vi "Import - Rx Packet.vi"(7 "Rx Packet":T1 {"Endianness" items=["big-endian"=0, "little-endian"=2]}, 8 "error in (no error)":errorcluster, 11 "Device Item Ref in":T6 format="%.0x") -> (0 "error out":errorcluster)   [LabVIEW 2016, in "UDP-Custom-Device System Explorer.lvlib"]
uses:
  UDP-Custom-Device System Explorer.lvlib
  <vilib>/NI Veristand/Custom Device API/Custom Device Item Ref.ctl
  Types/XML - New/ImpExp - Rx Packet Data.ctl
  <vilib>/NI Veristand/Custom Device API/Custom Device Item Info.ctl
  Shared/Types/Shared - Channel Data Type.ctl
  Shared/Types/Shared - Buffered.PacketInfo.ctl
  Shared/Types/Shared - Pointer Encoding.ctl
  <vilib>/NI Veristand/Custom Device API/Custom Device Channel.ctl
  <vilib>/NI Veristand/Custom Device API/Custom Device Channel Type.ctl
  Shared/Constants.vi
  Property Accessors/Shared Packet Accessors.lvlib
  Property Accessors/Rx Packet Accessors.lvlib
  <vilib>/NI VeriStand/Custom Device API/Custom Device API.lvlib
  Shared/UDP-Custom-Device Shared.lvlib
  Property Accessors/Rx Channel Accessors.lvlib
  Property Accessors/Rx Channel Section Accessors.lvlib
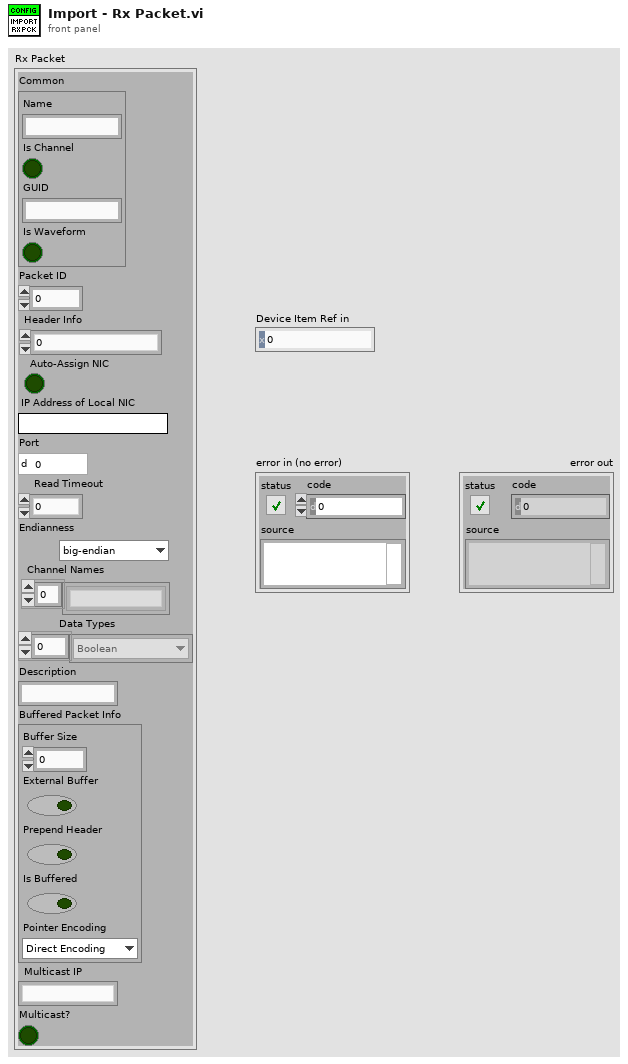
[diagram p1: front panel]
types:
  T1 = typedef "UDP-Custom-Device System Explorer.lvlib/ImpExp - Rx Packet Data.ctl" = cluster{"Common":T2, "Packet ID":i32, "Header Info":u32, "Auto-Assign NIC":bool, "IP Address of Local NIC":string, "Port":u16, "Read Timeout":i32, "Endianness":u16, "Channel Names":string[], "Data Types":T3[], "Description":string, "Buffered Packet Info":T4, "Multicast IP":string, "Multicast?":bool}
  T2 = typedef "Custom Device API.lvlib/Custom Device Item Info.ctl" = cluster{"Name":string, "Is Channel":bool, "GUID":string, "Is Waveform":bool}
  T3 = typedef "UDP-Custom-Device Shared.lvlib/Shared - Channel Data Type.ctl" = enum16{"Boolean", "Single", "Double", "I8", "I16", "I32", "I64", "U8", "U16", "U32", "U64"}
  T4 = typedef "UDP-Custom-Device Shared.lvlib/Shared - Buffered.PacketInfo.ctl" = cluster{"Buffer Size":i32, "External Buffer":bool, "Prepend Header":bool, "Is Buffered":bool, "Pointer Encoding":T5}
  T5 = typedef "UDP-Custom-Device Shared.lvlib/Shared - Pointer Encoding.ctl" = enum16{"Direct Encoding", "Conversion Encoding"}
  T6 = typedef "Custom Device API.lvlib/Custom Device Item Ref.ctl" = u64
  T7 = typedef "Custom Device API.lvlib/Custom Device Channel.ctl" = cluster{"Type":T8, "Units":string, "Default Value":dbl, "Faultable":bool, "Scalable":bool}
  T8 = typedef "Custom Device API.lvlib/Custom Device Channel Type.ctl" = enum16{"Input", "Output"}
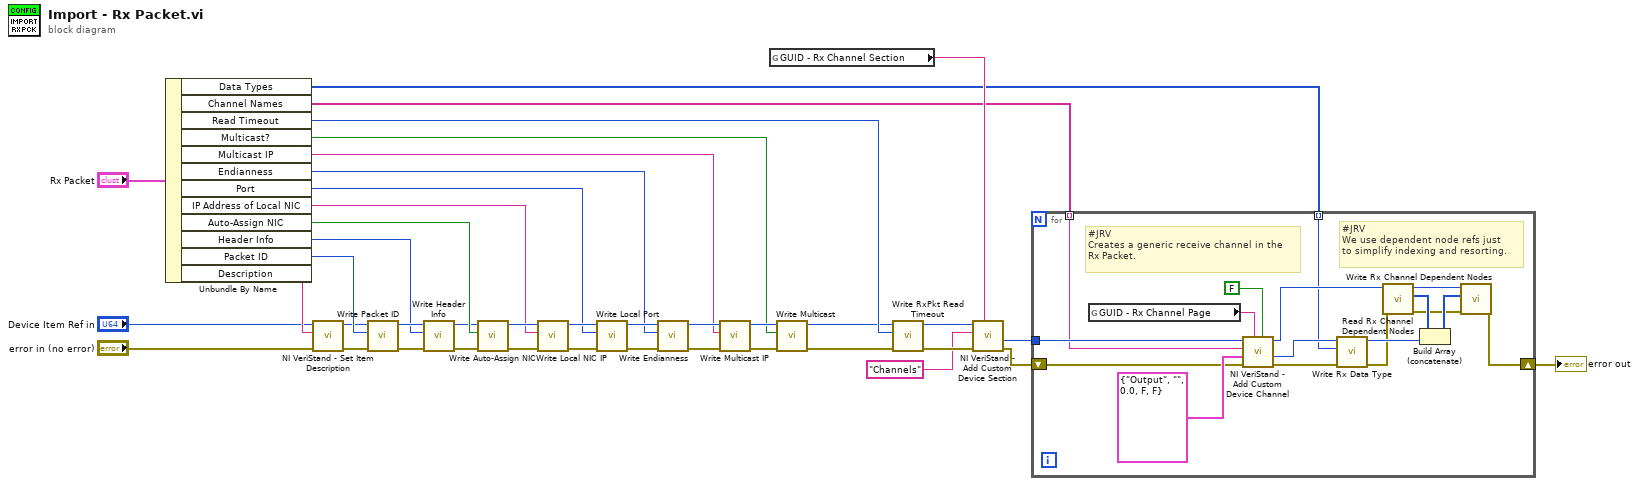
[diagram p0: block diagram]
diagram:
  n1 = Unbundle By Name("Rx Packet") -> ("Data Types"=w11:T3[], "Channel Names"=w10:string[], "Read Timeout"=w24:i32, "Multicast?"=w3:bool, "Multicast IP"=w4:string, "Endianness"=w25:u16, "Port"=w28:u16, "IP Address of Local NIC"=w31:string, "Auto-Assign NIC"=w35:bool, "Header Info"=w36:u32, "Packet ID"=w39:i32, "Description"=w22:string)
  n2 = call <vilib>:"NI VeriStand - Set Item Description.vi"("error in (no error)"="error in (no error)", "Description"=w22, "Item Ref in"="Device Item Ref in") -> ("error out"=w18:errorcluster, "Item Ref out"=w20:T6)  [unwired: 6 in, 1 out]
  n3 = call "Write Packet ID.vi"("error in (no error)"=w18, "Packet ID"=w39, "Node Ptr"=w20) -> ("error out"=w37:errorcluster, "Node Ptr out"=w38:T6)  [unwired: 7 in]
  n4 = call "Write Header Info.vi"("error in (no error)"=w37, "Header Info"=w36, "Node Ptr"=w38) -> ("error out"=w33:errorcluster, "Node Ptr out"=w34:T6)  [unwired: 7 in]
  n5 = call "Write Auto-Assign NIC.vi"("error in (no error)"=w33, "Auto-Assign NIC"=w35, "Node Ptr"=w34) -> ("error out"=w30:errorcluster, "Node Ptr out"=w32:T6)  [unwired: 7 in]
  n6 = call "Write Local NIC IP.vi"("error in (no error)"=w30, "IP Address of Local NIC"=w31, "Node Ptr"=w32) -> ("error out"=w27:errorcluster, "Node Ptr out"=w29:T6)  [unwired: 7 in]
  n7 = call "Write Local Port.vi"("error in (no error)"=w27, "Port"=w28, "Node Ptr"=w29) -> ("error out"=w23:errorcluster, "Node Ptr out"=w26:T6)  [unwired: 7 in]
  n8 = call "Write Endianness.vi"("error in (no error)"=w23, "Endianness"=w25, "Node Ptr"=w26) -> ("error out"=w6:errorcluster, "Node Ptr out"=w5:T6)  [unwired: 7 in]
  n9 = call "Write Multicast IP.vi"("error in (no error)"=w6, "Multicast IP Address"=w4, "Node Ptr"=w5) -> ("error out"=w8:errorcluster, "Node Ptr out"=w7:T6)  [unwired: 7 in]
  n10 = global read "Constants.vi" "GUID - Rx Channel Section"() -> (w14:string)
  n11 = call "Write Multicast.vi"("error in (no error)"=w8, "Multicast"=w3, "Node Ptr"=w7) -> ("error out"=w1:errorcluster, "Node Ptr out"=w2:T6)  [unwired: 7 in]
  n12 = call "Write RxPkt Read Timeout.vi"("error in (no error)"=w1, "Read Timeout"=w24, "Node Ptr"=w2) -> ("error out"=w16:errorcluster, "Node Ptr out"=w17:T6)  [unwired: 7 in]
  n13 = call <vilib>:"NI VeriStand - Add Custom Device Section.vi"("GUID (Default Section)"=w14, "error in (no error)"=w16, "Section Name"="Channels", "Parent Ref in"=w17) -> ("error out"=w12:errorcluster, "Section Ptr"=w13:T6)  [unwired: 4 in, 2 out]
  n14 = for {
    tunnel: w13 -> [w45]
    tunnel: w11 -> [w43] mode=indexing
    tunnel: w10 -> [w42] mode=indexing
    shift-right: [w41] -> w9
    shift-left: w12 -> [w44]
    # "#JRV\nWe use dependent node refs just\nto simplify indexing and resorting."
    # "#JRV\nCreates a generic receive channel in the \nRx Packet."
    n15 = global read "Constants.vi" "GUID - Rx Channel Page"() -> (w57:string)
    n16 = call <vilib>:"NI VeriStand - Add Custom Device Channel.vi"("Highlight? (F)"=FALSE, "GUID (Default Channel)"=w57, "error in (no error)"=w44, "Channel"=T7 {"Type"=enum."Output", "Units"="", "Default Value"=0.0, "Faultable"=FALSE, "Scalable"=FALSE}, "Channel Name"=w42, "Parent Ref in"=w45) -> ("error out"=w53:errorcluster, "Channel Ref"=w54:T6, "Parent Ref out"=w51:T6)  [unwired: 2 in, 1 out]
    n17 = call "Write Rx Data Type.vi"("error in (no error)"=w53, "Data Type"=w43, "Node Ptr"=w54) -> ("error out"=w50:errorcluster, "Node Ptr out"=w52:T6)  [unwired: 7 in]
    n18 = call "Read Rx Channel Dependent Nodes.vi"("error in (no error)"=w50, "Node Ptr"=w51) -> ("error out"=w46:errorcluster, "Dependent Node Refs"=w48:T6[], "Node Ptr out"=w49:T6)  [unwired: 7 in]
    n19 = Build Array (concatenate)(w48, w52) -> (w47:T6[])
    n20 = call "Write Rx Channel Dependent Nodes.vi"("error in (no error)"=w46, "Dependent Node Refs"=w47, "Node Ptr"=w49) -> ("error out"=w41:errorcluster)  [unwired: 7 in, 1 out]
  }
  "error out" <- w9
